vi "S2C_CMD_FindValue.vi"(8 "Error In":errorcluster, 9 "Row":i32, 10 "CtlRef":refnum<vi>, 11 "ItemTag":string) -> (0 "Error Out":errorcluster, 2 "Found?":bool, 3 "Value_Int":string)   [LabVIEW 2015]
doc: "Finds the Int value for a selected command type."
uses:
  S2C_CMD_Globals.vi
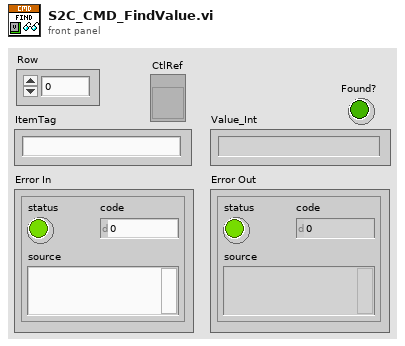
[diagram p1: front panel]
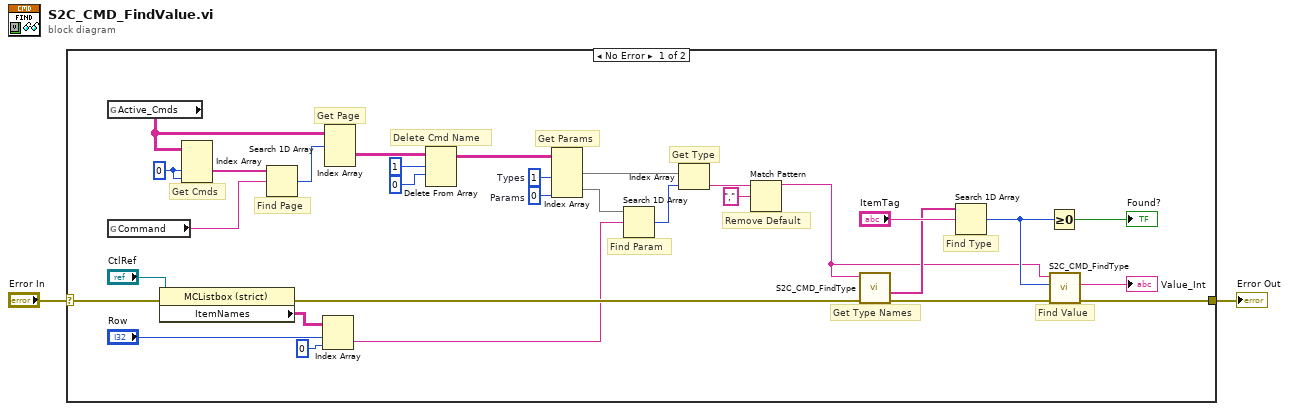
[diagram p0: block diagram]
diagram:
  n1 = case shown="No Error" "Error In" {
    selector: "Error In" -> [w33 w34]
    tunnel: [w27 w34] -> w1
    frame No Error {
      w20 = 0  # Params
      w21 = 1  # Types
      w24 = 0 ("disabled index (row)")
      # "Delete Cmd Name"
      # "Remove Default"
      # "Find Value"
      # "Find Type"
      # "Get Type Names"
      # "Get Type"
      # "Find Param"
      # "Get Params"
      # "Get Page"
      # "Find Page"
      # "Get Cmds"
      n2 = global read "S2C_CMD_Globals.vi" "Active_Cmds"() -> (w23:string[][][])
      n3 = global read "S2C_CMD_Globals.vi" "Command"() -> (w11:string)
      n4 = property class="MCListbox (strict)"(reference="CtlRef", error in=w33) -> (error out=w28:errorcluster, "ItemNames"=w31:string[][])  [unwired: 1 out]
      n5 = Index Array(array=w23, index (dim 1)=w24, index (dim 2)=w24) -> (element=w25:string[])  [unwired: 1 in]
      n6 = Search 1D Array(1D array=w25, element=w11) -> (index of element=w22:i32)  [unwired: 1 in]
      n7 = Index Array(array=w31, index (row)="Row", index (col)=0 ("disabled index (col)")) -> (element=w10:string)
      n8 = Index Array(array=w23, index (dim 0)=w22) -> (element=w6:string[][])  [unwired: 2 in]
      n9 = Delete From Array(array=w6, length=1, index (row)=0) -> (array with subset deleted=w5:string[][])  [unwired: 1 in, 1 out]
      n10 = Index Array(array=w5, index (col) #1=w21, index (col) #2=w20) -> (element #1=w18:string[], element #2=w19:string[])  [unwired: 2 in]
      n11 = Search 1D Array(1D array=w19, element=w10) -> (index of element=w17:i32)  [unwired: 1 in]
      n12 = Index Array(array=w18, index=w17) -> (element=w9:string)
      n13 = Match Pattern(string=w9, regular expression=",") -> (before substring=w7:string)  [unwired: 1 in, 3 out]
      n14 = call "S2C_CMD_FindType.vi"("Error In"=w28, "TypeString"=w7) -> ("Error Out"=w13:errorcluster, "AllValues"=w14:string[])  [unwired: 5 in, 3 out]
      n15 = Search 1D Array(1D array=w14, element="ItemTag") -> (index of element=w12:i32)  [unwired: 1 in]
      n16 = Greater Or Equal To 0?(x=w12) -> (x >= 0?=→"Found?":bool)
      n17 = call "S2C_CMD_FindType.vi"("Error In"=w13, "Index"=w12, "TypeString"=w7) -> ("Error Out"=w27:errorcluster, "Value_Int"=→"Value_Int":string)  [unwired: 4 in, 3 out]
    }
    frame Error {
    }
  }
  "Error Out" <- w1
